vi "Grabu32.vi"(9 "byte order":T1(ring)=enum."little-endian", 11 "String in":string) -> (2 "Value":u32, 3 "String out":string)   [LabVIEW 2022 SP3]
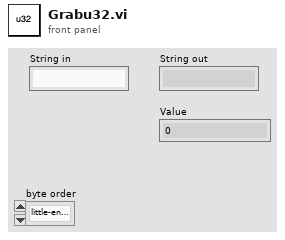
[diagram p1: front panel]
types:
  T1 = enum16{"big-endian, network order", "native, host order", "little-endian"}
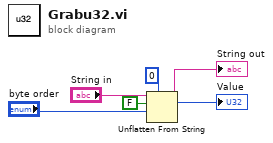
[diagram p0: block diagram]
diagram:
  n1 = Unflatten From String(type=u32 0 ("offset (0)"), binary string="String in", data includes array or string size? (T)=FALSE, byte order (0:big-endian, network order)="byte order") -> (rest of the binary string=→"String out":string, value=→"Value":u32)  [unwired: 1 in, 1 out]
